vi "PH_AxisGUI_NF2.evt Call Width Axis 2.vi"(0 "i ref in":refnum<vi>, 1 "NF GUI 2 instance":string, 2 "Width Axis 1":i32 caption="Width Axis 2", 5 "error in":errorcluster) -> (14 "i ref out":refnum<vi>, 19 "error out":errorcluster)   [LabVIEW 2014, in "PH_AxisGUI_NF2.lvlib"]
uses:
  PH_AxisGUI_NF2.lvlib
  CS_Core/CSSystem/CoreLib/CoreLib.int 2 byte array.vi
  CS_Core/CSSystem/CoreLib/CoreLib.lvlib
  CS_Core/BaseProcess/BaseProcess.lvlib
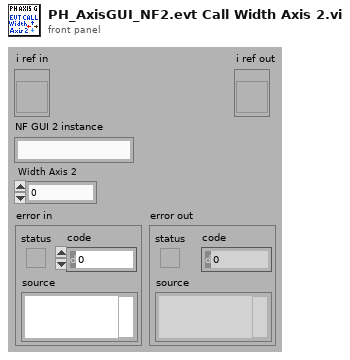
[diagram p1: front panel]
types:
  T1 = typedef "CoreDefs.rawDataType.ctl" = i8[]
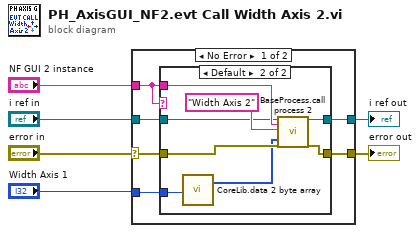
[diagram p0: block diagram]
diagram:
  n1 = case shown="No Error" "error in" {
    selector: "error in" -> [w8 w23]
    tunnel: [w12 w23] -> w3
    tunnel: "NF GUI 2 instance" -> [w7 _]
    tunnel: "i ref in" -> [w11 w24]
    tunnel: [w10 w24] -> w5
    tunnel: "Width Axis 1" -> [w9 _]
    frame No Error {
      n2 = case shown="Default" w7 {
        tunnel: [w14 w22] -> w12
        tunnel: w7 -> [_ w20]
        tunnel: w8 -> [w14 w19]
        tunnel: w11 -> [w13 w18]
        tunnel: [w13 w17] -> w10
        tunnel: w9 -> [_ w16]
        frame "N/A" {
        }
        frame Default {
          n3 = call-poly "CoreLib.data 2 byte array.vi"("i32"=w16) -> ("byteArray out"=w15:T1)  [unwired: 18 in]
          n4 = call "BaseProcess.call process 2.vi"("i ref in"=w18, "Object"=w20, "Selector"="Width Axis 2", "Data"=w15, "error in (no error)"=w19) -> ("i ref out"=w17:refnum<vi>, "error out"=w22:errorcluster)  [unwired: 13 in]
        }
      }
    }
    frame Error {
    }
  }
  "i ref out" <- w5
  "error out" <- w3
